vi "Get Data Size.vi"(8 "error in (no error)":errorcluster, 11 "Composite Object in":refnum<class "CConfig Object.lvclass">) -> (0 "error out":errorcluster, 2 "Elements":i32, 3 "Composite Object out":refnum<class "CConfig Object.lvclass">)   [LabVIEW 2013, in "CConfig Object.lvclass"]
doc: "Copyright 2018, Carya Automatisering, Wiebe Walstra."
uses:
  CConfig Object.lvclass
  CConfig Object.lvclass/CConfig Object.ctl
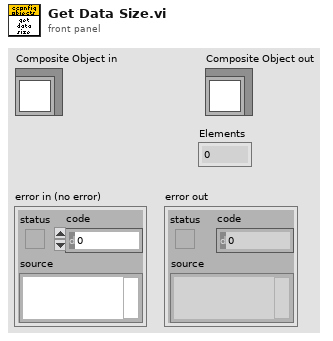
[diagram p1: front panel]
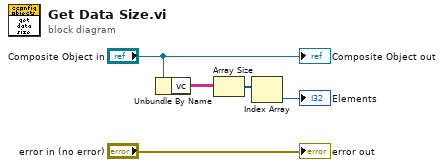
[diagram p0: block diagram]
diagram:
  n1 = Unbundle By Name("Composite Object in") -> ("vc"=w3:string[][])
  n2 = Array Size(array=w3) -> (size(s)=w2:i32[])
  n3 = Index Array(array=w2) -> (element=→"Elements":i32)  [unwired: 1 in]
  "error out" <- "error in (no error)"
  "Composite Object out" <- "Composite Object in"
